vi "Autonomous Independent.vi"   [LabVIEW 2015]
doc: "This VI is called when autonomous begins, and will automatically be terminated when autonomous ends. You can carry out timed or sensor driven robot movement independently without needing to return to the caller."
uses:
  <vilib>/Rock Robotics/WPI/Solenoid/WPI_SolenoidValue.ctl
  <vilib>/Rock Robotics/WPI/Utilities/WPI_GetSetVariantRefNum.vi
  <vilib>/Rock Robotics/Network Tables/NT Read String.vi
  <vilib>/Rock Robotics/Network Tables/NT Read Number.vi
  <vilib>/Rock Robotics/WPI/Solenoid/WPI_SolenoidSetEnum.vi
  <vilib>/Rock Robotics/Network Tables/NT Write Numeric Array.vi
panel:
  # "Be sure to right-click and choose Data Operations>>Make Current Value default if you want to save the array values with the VI"
types:
  T1 = typedef "WPI_JoystickDevRef.ctl" = cluster{"Device":T2}
  T2 = typedef "WPI_JoystickDeviceEnum.ctl" = enum16{"USB 0", "USB 1", "USB 2", "USB 3", "USB 4", "USB 5"}
  T3 = typedef "WPI_ServoDeviceRef.ctl" = cluster{"DeviceStatus":errorcluster, "PWM Channel":T4, "DeadBand":T5}
  T4 = typedef "FPGA_DIOPWMChannel.ctl" = enum8{"PWM 0", "PWM 1", "PWM 2", "PWM 3", "PWM 4", "PWM 5", "PWM 6", "PWM 7", "PWM 8", "PWM 9", "PWM MXP 0", "PWM MXP 1", "PWM MXP 2", "PWM MXP 3", "PWM MXP 4", "PWM MXP 5", "PWM MXP 6", "PWM MXP 7", "PWM MXP 8", "PWM MXP 9", "Invalid"}
  T5 = typedef "WPI_PWMDeadband.ctl" = cluster{"Name":string, "maxPositivePwm":i32, "minPositivePwm":i32, "centerPwm":i32, "maxNegativePwm":i32, "minNegativePwm":i32, "angularRange":u16}
  T6 = typedef "WPI_SolenoidValue.ctl" = enum16{"Off", "On", "Forward", "Reverse"}
  T7 = typedef "WPI_SwitchDevRef.ctl" = cluster{"DevStatus":errorcluster, "DIO Channel":T8, "CntIndex":T9, "Normally Closed":bool}
  T8 = typedef "FPGA_DIOChannel.ctl" = enum8{"DIO 0", "DIO 1", "DIO 2", "DIO 3", "DIO 4", "DIO 5", "DIO 6", "DIO 7", "DIO 8", "DIO 9", "DIO MXP 0", "DIO MXP 1", "DIO MXP 2", "DIO MXP 3", "DIO MXP 4", "DIO MXP 5", "DIO MXP 6", "DIO MXP 7", "DIO MXP 8", "DIO MXP 9", "DIO MXP 10", "DIO MXP 11", "DIO MXP 12", "DIO MXP 13", "DIO MXP 14", "DIO MXP 15", "Invalid"}
  T9 = typedef "FPGA_CounterCtrSystemIndex.ctl" = enum8{"Ctr 0", "Ctr 1", "Ctr 2", "Ctr 3", "Ctr 4", "Ctr 5", "Ctr 6", "Ctr 7", "Invalid"}
  T10 = typedef "WPI_SolenoidDevRef.ctl" = cluster{"DevStatus":errorcluster, "Pneumatics Control Module":u8, "Forward Solenoid Channel":T11, "Reverse Solenoid Channel":T11}
  T11 = typedef "WPI_SolenoidChannel.ctl" = enum8{"Solenoid 0", "Solenoid 1", "Solenoid 2", "Solenoid 3", "Solenoid 4", "Solenoid 5", "Solenoid 6", "Solenoid 7", "Invalid"}
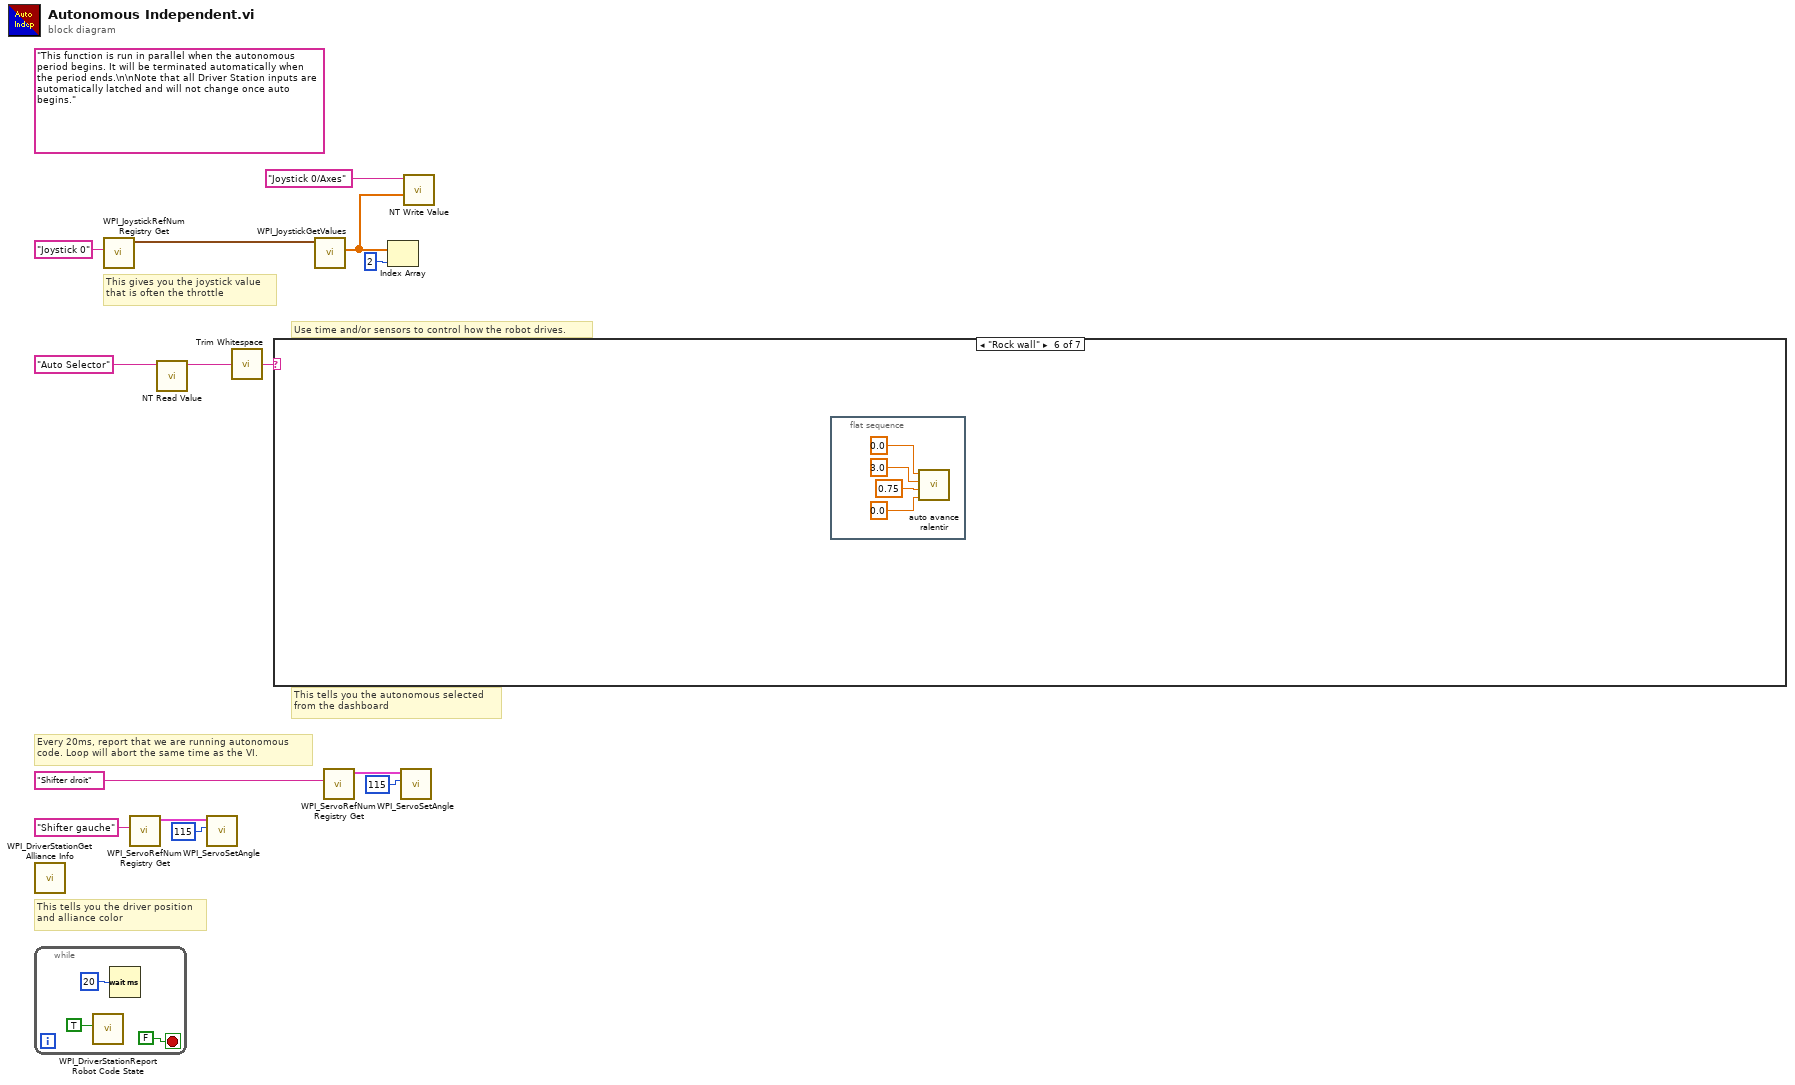
[diagram p0: block diagram]
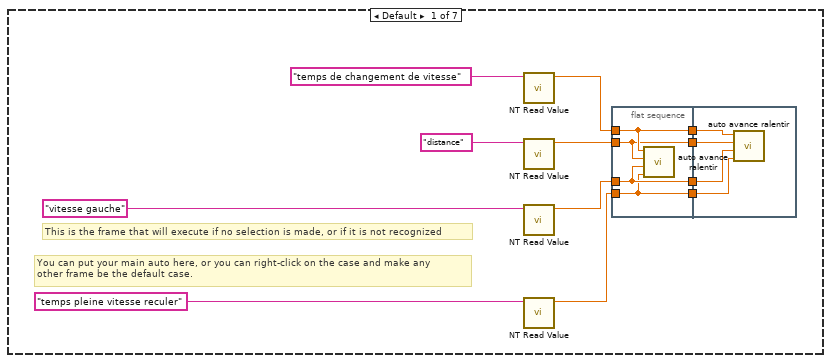
[diagram p2: hidden frame]
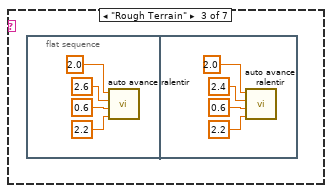
[diagram p4: hidden frame]
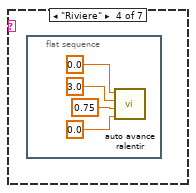
[diagram p5: hidden frame]
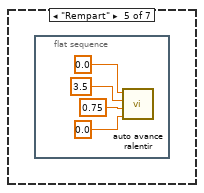
[diagram p6: hidden frame]
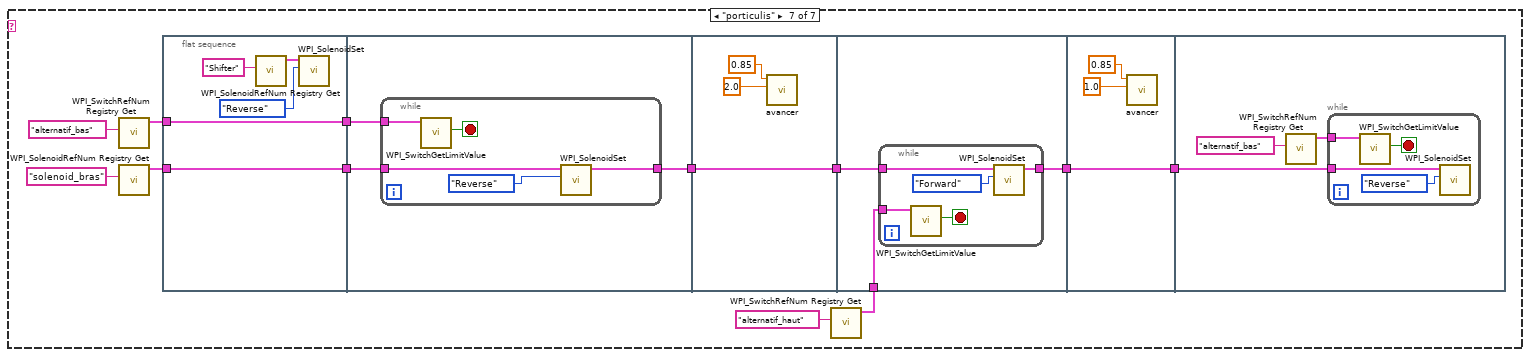
[diagram p7: hidden frame]
diagram:
  (unwired) "This function is run in parallel when the autonomous period begins. It will be terminated automatically when the period ends.\n\nNote that all Driver Station inputs are automatically latched and will not change once auto begins."
  # "This tells you the autonomous selected\nfrom the dashboard"
  # "Every 20ms, report that we are running autonomous\ncode. Loop will abort the same time as the VI."
  # "This gives you the joystick value\nthat is often the throttle"
  # "Use time and/or sensors to control how the robot drives."
  # "This tells you the driver position\nand alliance color"
  n1 = call <vilib>:"WPI_DriverStationGet Alliance Info.vi"() -> ()  [unwired: 12 out]
  n2 = while {
    stop <- FALSE stop-if-true
    n3 = call <vilib>:"WPI_DriverStationReport Robot Code State.vi"("Autonomous"=TRUE) -> ()  [unwired: 10 in, 1 out]
    n4 = Wait (ms)(milliseconds to wait=u32 20) -> ()  [unwired: 1 out]
  }
  n5 = call <vilib>:"WPI_JoystickRefNum Registry Get.vi"("refnum name"="Joystick 0") -> ("JoystickDevRef"=w13:T1)  [unwired: 1 in, 9 out]
  n6 = call <vilib>:"WPI_ServoRefNum Registry Get.vi"("refnum name"="Shifter gauche") -> ("ServoDeviceRef"=w3:T3)  [unwired: 9 in, 1 out]
  n7 = call-poly <vilib>:"NT Read Value.vi"("Name"="Auto Selector") -> ("String"=w1:string)  [unwired: 9 in, 1 out]
  n8 = call <vilib>:"WPI_ServoSetAngle.vi"("Angle"=115, "ServoDeviceRef"=w3) -> ()  [unwired: 8 in, 2 out]
  n9 = call <vilib>:"Trim Whitespace.vi"("string"=w1) -> ("trimmed string"=w2:string)  [unwired: 1 in]
  n10 = case shown="\"Rock wall\"" w2 {
    frame Default {
      # "You can put your main auto here, or you can right-click on the case and make any\nother frame be the default case."
      # "This is the frame that will execute if no selection is made, or if it is not recognized"
      n11 = call-poly <vilib>:"NT Read Value.vi"("Name"="temps de changement de vitesse") -> ("Numeric"=w22:dbl)  [unwired: 9 in, 1 out]
      n12 = call-poly <vilib>:"NT Read Value.vi"("Name"="distance") -> ("Numeric"=w23:dbl)  [unwired: 9 in, 1 out]
      n13 = call-poly <vilib>:"NT Read Value.vi"("Name"="vitesse gauche") -> ("Numeric"=w24:dbl)  [unwired: 9 in, 1 out]
      n14 = call-poly <vilib>:"NT Read Value.vi"("Name"="temps pleine vitesse reculer") -> ("Numeric"=w25:dbl)  [unwired: 9 in, 1 out]
      n15 = flat-sequence {
        tunnel: w22 -> [w33]
        tunnel: w24 -> [w31]
        tunnel: w25 -> [w30]
        tunnel: w23 -> [w32]
        tunnel: [w33] -> w21
        tunnel: [w32] -> w20
        tunnel: [w31] -> w19
        tunnel: [w30] -> w18
        tunnel: w21 -> [w37]
        tunnel: w20 -> [w36]
        tunnel: w19 -> [w35]
        tunnel: w18 -> [w34]
        frame #0 {
          n16 = call "auto avance ralentir.vi"("Temps reculer"=w30, "vitesse gauche"=w31, "temps avancer"=w32, "temps de changement de direction"=w33) -> ()  [unwired: 8 in]
        }
        frame #1 {
          n17 = call "auto avance ralentir.vi"("Temps reculer"=w34, "vitesse gauche"=w35, "temps avancer"=w36, "temps de changement de direction"=w37) -> ()  [unwired: 8 in]
        }
      }
    }
    frame "rien" {
    }
    frame "Rough Terrain" {
      n18 = flat-sequence {
        frame #0 {
          n19 = call "auto avance ralentir.vi"("Temps reculer"=2.2, "vitesse gauche"=0.6, "temps avancer"=2.6, "temps de changement de direction"=2.0) -> ()  [unwired: 8 in]
        }
        frame #1 {
          n20 = call "auto avance ralentir.vi"("Temps reculer"=2.2, "vitesse gauche"=0.6, "temps avancer"=2.4, "temps de changement de direction"=2.0) -> ()  [unwired: 8 in]
        }
      }
    }
    frame "Riviere" {
      n21 = flat-sequence {
        frame #0 {
          n22 = call "auto avance ralentir.vi"("Temps reculer"=0.0, "vitesse gauche"=0.75, "temps avancer"=3.0, "temps de changement de direction"=0.0) -> ()  [unwired: 8 in]
        }
      }
    }
    frame "Rempart" {
      n23 = flat-sequence {
        frame #0 {
          n24 = call "auto avance ralentir.vi"("Temps reculer"=0.0, "vitesse gauche"=0.75, "temps avancer"=3.5, "temps de changement de direction"=0.0) -> ()  [unwired: 8 in]
        }
      }
    }
    frame "Rock wall" {
      n25 = flat-sequence {
        frame #0 {
          n26 = call "auto avance ralentir.vi"("Temps reculer"=0.0, "vitesse gauche"=0.75, "temps avancer"=3.0, "temps de changement de direction"=0.0) -> ()  [unwired: 8 in]
        }
      }
    }
    frame "porticulis" {
      n27 = call <vilib>:"WPI_SwitchRefNum Registry Get.vi"("refnum name"="alternatif_bas") -> ("SwitchDevRef"=w69:T7)  [unwired: 9 in, 1 out]
      n28 = call <vilib>:"WPI_SolenoidRefNum Registry Get.vi"("refnum name"="solenoid_bras") -> ("SolenoidDevRef"=w66:T10)  [unwired: 9 in, 1 out]
      n29 = flat-sequence {
        tunnel: w66 -> [w73]
        tunnel: w69 -> [w74]
        tunnel: [w74] -> w60
        tunnel: [w73] -> w59
        tunnel: [w75] -> w63
        tunnel: w60 -> [w77]
        tunnel: w59 -> [w76]
        tunnel: [w85] -> w64
        tunnel: w63 -> [w85]
        tunnel: w67 -> [w88]
        tunnel: w64 -> [w87]
        tunnel: [w86] -> w62
        tunnel: w62 -> [w96]
        tunnel: [w96] -> w61
        tunnel: w61 -> [w99]
        frame #0 {
          n30 = call <vilib>:"WPI_SolenoidRefNum Registry Get.vi"("refnum name"="Shifter") -> ("SolenoidDevRef"=w72:T10)  [unwired: 9 in, 1 out]
          n31 = call-poly <vilib>:"WPI_SolenoidSet.vi"("Value"=WPI_SolenoidValue."Reverse", "SolenoidDevRef"=w72) -> ()  [unwired: 8 in, 2 out]
        }
        frame #1 {
          n32 = while {
            tunnel: w77 -> [w82]
            tunnel: w76 -> [w80]
            tunnel: [w78] -> w75
            stop <- w81 stop-if-true
            n33 = call <vilib>:"WPI_SwitchGetLimitValue.vi"("SwitchDevRef"=w82) -> ("Switch Pressed"=w81:bool)  [unwired: 8 in, 2 out]
            n34 = call-poly <vilib>:"WPI_SolenoidSet.vi"("Value"=WPI_SolenoidValue."Reverse", "SolenoidDevRef"=w80) -> ("SolenoidDevRef"=w78:T10)  [unwired: 8 in, 1 out]
          }
        }
        frame #2 {
          n35 = call "avancer.vi"("Distance"=2.0, "Vitesse"=0.85) -> ()  [unwired: 10 in]
        }
        frame #3 {
          n36 = while {
            tunnel: w88 -> [w93]
            tunnel: w87 -> [w91]
            tunnel: [w89] -> w86
            stop <- w92 stop-if-true
            n37 = call <vilib>:"WPI_SwitchGetLimitValue.vi"("SwitchDevRef"=w93) -> ("Switch Pressed"=w92:bool)  [unwired: 8 in, 2 out]
            n38 = call-poly <vilib>:"WPI_SolenoidSet.vi"("Value"=WPI_SolenoidValue."Forward", "SolenoidDevRef"=w91) -> ("SolenoidDevRef"=w89:T10)  [unwired: 8 in, 1 out]
          }
        }
        frame #4 {
          n39 = call "avancer.vi"("Distance"=1.0, "Vitesse"=0.85) -> ()  [unwired: 10 in]
        }
        frame #5 {
          n40 = call <vilib>:"WPI_SwitchRefNum Registry Get.vi"("refnum name"="alternatif_bas") -> ("SwitchDevRef"=w98:T7)  [unwired: 9 in, 1 out]
          n41 = while {
            tunnel: w99 -> [w103]
            tunnel: w98 -> [w100]
            stop <- w101 stop-if-true
            n42 = call <vilib>:"WPI_SwitchGetLimitValue.vi"("SwitchDevRef"=w100) -> ("Switch Pressed"=w101:bool)  [unwired: 8 in, 2 out]
            n43 = call-poly <vilib>:"WPI_SolenoidSet.vi"("Value"=WPI_SolenoidValue."Reverse", "SolenoidDevRef"=w103) -> ()  [unwired: 8 in, 2 out]
          }
        }
      }
      n44 = call <vilib>:"WPI_SwitchRefNum Registry Get.vi"("refnum name"="alternatif_haut") -> ("SwitchDevRef"=w67:T7)  [unwired: 9 in, 1 out]
    }
  }
  n45 = call <vilib>:"WPI_JoystickGetValues.vi"("JoystickDevRef"=w13) -> ("Axes"=w10:dbl[])  [unwired: 6 in, 4 out]
  n46 = call <vilib>:"WPI_ServoRefNum Registry Get.vi"("refnum name"="Shifter droit") -> ("ServoDeviceRef"=w5:T3)  [unwired: 9 in, 1 out]
  n47 = Index Array(array=w10, index=2) -> ()  [unwired: 1 out]
  n48 = call <vilib>:"WPI_ServoSetAngle.vi"("Angle"=115, "ServoDeviceRef"=w5) -> ()  [unwired: 8 in, 2 out]
  n49 = call-poly <vilib>:"NT Write Value.vi"("Numeric Array"=w10, "Name"="Joystick 0/Axes") -> ()  [unwired: 9 in, 1 out]
